vi "Manual - Invert(FGV).vi"(7 "Action":T1=enum."Write", 8 "error in (no error)":errorcluster, 11 "invert in":bool=TRUE) -> (0 "error out":errorcluster, 3 "invert out":bool)   [LabVIEW 2019]
uses:
  Controls/FGV States.ctl
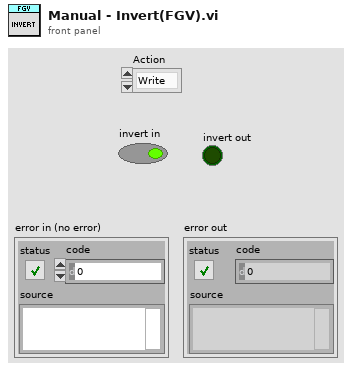
[diagram p1: front panel]
types:
  T1 = typedef "FGV States.ctl" = enum16{"Read", "Write"}
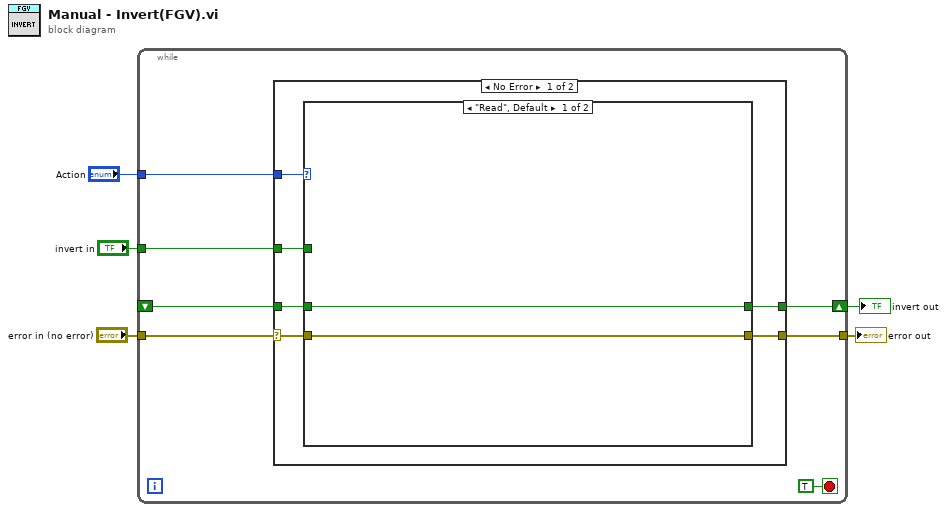
[diagram p0: block diagram]
diagram:
  n1 = while {
    tunnel: "Action" -> [w12]
    tunnel: "error in (no error)" -> [w10]
    tunnel: [w9] -> w3
    tunnel: "invert in" -> [w8]
    shift-right: [w7] -> w1
    shift-left: _ -> [w6]
    stop <- TRUE stop-if-true
    n2 = case shown="No Error" w10 {
      selector: w10 -> [w16 w24]
      tunnel: w12 -> [w18 _]
      tunnel: [w17 w24] -> w9
      tunnel: w8 -> [w15 _]
      tunnel: [w14 w23] -> w7
      tunnel: w6 -> [w13 w23]
      frame No Error {
        n3 = case shown="\"Read\", Default" w18 {
          tunnel: [w20 w22] -> w17
          tunnel: w16 -> [w20 w22]
          tunnel: w15 -> [_ w21]
          tunnel: [w19 w21] -> w14
          tunnel: w13 -> [w19 _]
          frame "Read", Default {
          }
          frame "Write" {
          }
        }
      }
      frame Error {
      }
    }
  }
  "error out" <- w3
  "invert out" <- w1
